vi "Actor Core.vi"(8 "error in":errorcluster, 11 "TCP_Server in":refnum<class "TCP_Server.lvclass">) -> (0 "error out":errorcluster, 3 "Actor out":refnum<class "Actor.lvclass">)   [LabVIEW 2023, in "TCP_Server.lvlib" / "TCP_Server.lvclass"]
doc: "(<B>Filename</B>: Actor Framework.lvlib:Actor.lvclass:Actor Core.vi)\n\nReceives messages to the actor, reacts to them, and initiates any error handling that may shut the actor down.\n\nDescendant classes may override this VI to append parallel tasks for the actor to complete while it handles messages. Overrides use the Call Parent Class Method node."
uses:
  TCP_Server.lvclass
  <vilib>/ActorFramework/Actor/Actor.lvclass
  TCP_Server.lvclass/TCP_Server.ctl
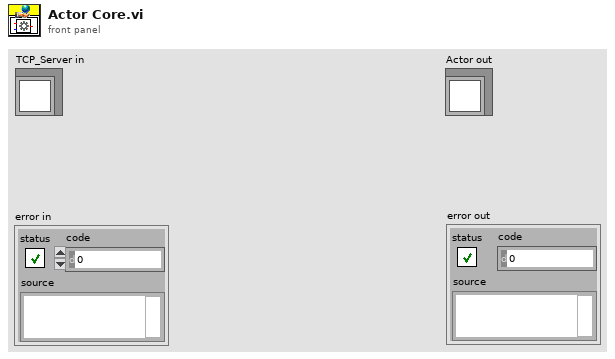
[diagram p1: front panel]
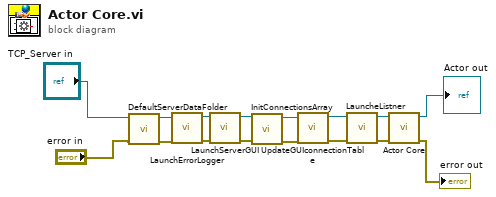
[diagram p0: block diagram]
diagram:
  n1 = call "DefaultServerDataFolder.vi"("error in (no error)"="error in", "TCP_Server in"="TCP_Server in") -> ("error out"=w4:errorcluster, "TCP_Server out"=w3:refnum<class "TCP_Server.lvclass">)  [unwired: 8 in]
  n2 = call "LaunchErrorLogger.vi"("error in (no error)"=w4, "TCP_Server in"=w3) -> ("error out"=w12:errorcluster, "TCP_Server out"=w10:refnum<class "TCP_Server.lvclass">)  [unwired: 8 in]
  n3 = call "LaunchServerGUI.vi"("error in (no error)"=w12, "TCP_Server in"=w10) -> ("error out"=w11:errorcluster, "TCP_Server out"=w9:refnum<class "TCP_Server.lvclass">)  [unwired: 8 in]
  n4 = call "InitConnectionsArray.vi"("error in (no error)"=w11, "TCP_Server in"=w9) -> ("error out"=w8:errorcluster, "TCP_Server out"=w6:refnum<class "TCP_Server.lvclass">)  [unwired: 8 in]
  n5 = call "UpdateGUIconnectionTable.vi"("error in (no error)"=w8, "TCP_Server in"=w6) -> ("error out"=w7:errorcluster, "TCP_Server out"=w5:refnum<class "TCP_Server.lvclass">)  [unwired: 8 in]
  n6 = call "LauncheListner.vi"("error in (no error)"=w7, "TCP_Server in"=w5) -> ("error out"=w13:errorcluster, "TCP_Server out"=w14:refnum<class "TCP_Server.lvclass">)  [unwired: 8 in]
  n7 = call-parent "Actor Core.vi"("error in"=w13, "Actor in"=w14) -> ("error out"=→"error out":errorcluster, "Actor out"=→"Actor out":refnum<class "Actor.lvclass">)  [unwired: 8 in]
